vi "DUT Test.vi"(8 "error in (no error)":errorcluster, 11 "DUT cluster in":T1) -> (0 "error out":errorcluster, 3 "DUT cluster out":T1)   [LabVIEW 2018, in "Application.lvlib"]
uses:
  Application.lvlib
  DRV cluster.ctl
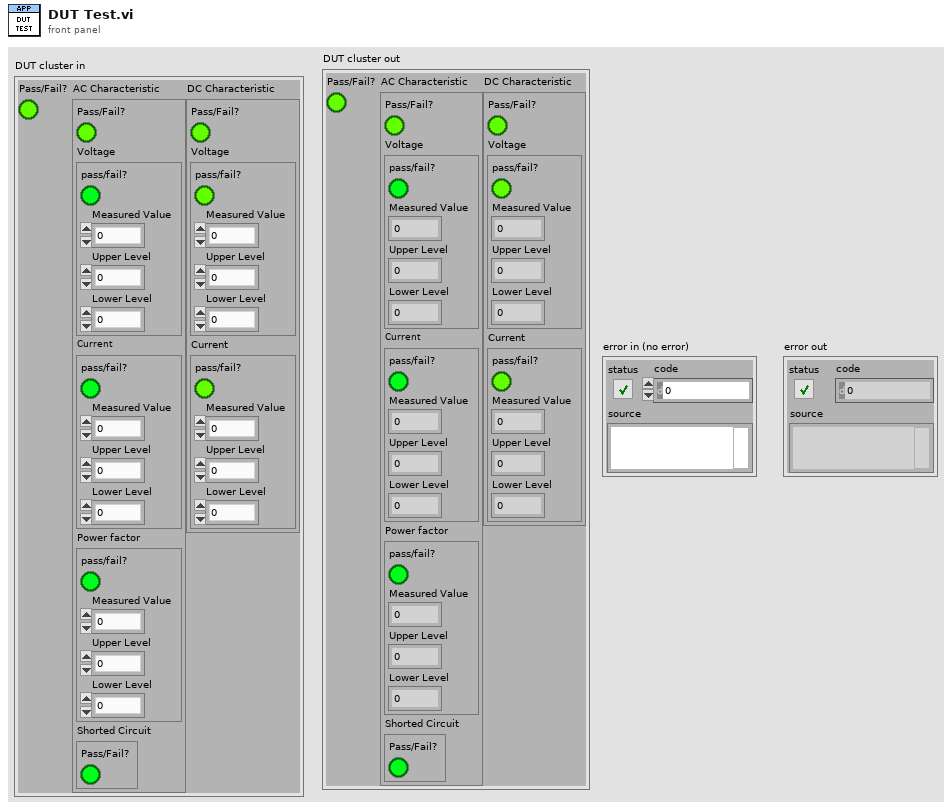
[diagram p1: front panel]
types:
  T1 = typedef "Application.lvlib/DRV cluster.ctl" = cluster{"Pass/Fail?":bool, "AC Characteristic":cluster{"Pass/Fail?":bool, "Voltage":cluster{"pass/fail?":bool, "Measured Value":dbl, "Upper Level":dbl, "Lower Level":dbl}, "Current":cluster{"pass/fail?":bool, "Measured Value":dbl, "Upper Level":dbl, "Lower Level":dbl}, "Power factor":cluster{"pass/fail?":bool, "Measured Value":dbl, "Upper Level":dbl, "Lower Level":dbl}, "Shorted Circuit":cluster{"Pass/Fail?":bool}}, "DC Characteristic":cluster{"Pass/Fail?":bool, "Voltage":cluster{"pass/fail?":bool, "Measured Value":dbl, "Upper Level":dbl, "Lower Level":dbl}, "Current":cluster{"pass/fail?":bool, "Measured Value":dbl, "Upper Level":dbl, "Lower Level":dbl}}}
  T2 = cluster{"Pass/Fail?":bool, "Voltage":cluster{"pass/fail?":bool, "Measured Value":dbl, "Upper Level":dbl, "Lower Level":dbl}, "Current":cluster{"pass/fail?":bool, "Measured Value":dbl, "Upper Level":dbl, "Lower Level":dbl}}
  T3 = cluster{"Pass/Fail?":bool, "Voltage":cluster{"pass/fail?":bool, "Measured Value":dbl, "Upper Level":dbl, "Lower Level":dbl}, "Current":cluster{"pass/fail?":bool, "Measured Value":dbl, "Upper Level":dbl, "Lower Level":dbl}, "Power factor":cluster{"pass/fail?":bool, "Measured Value":dbl, "Upper Level":dbl, "Lower Level":dbl}, "Shorted Circuit":cluster{"Pass/Fail?":bool}}
  T4 = cluster{"pass/fail?":bool, "Measured Value":dbl, "Upper Level":dbl, "Lower Level":dbl}
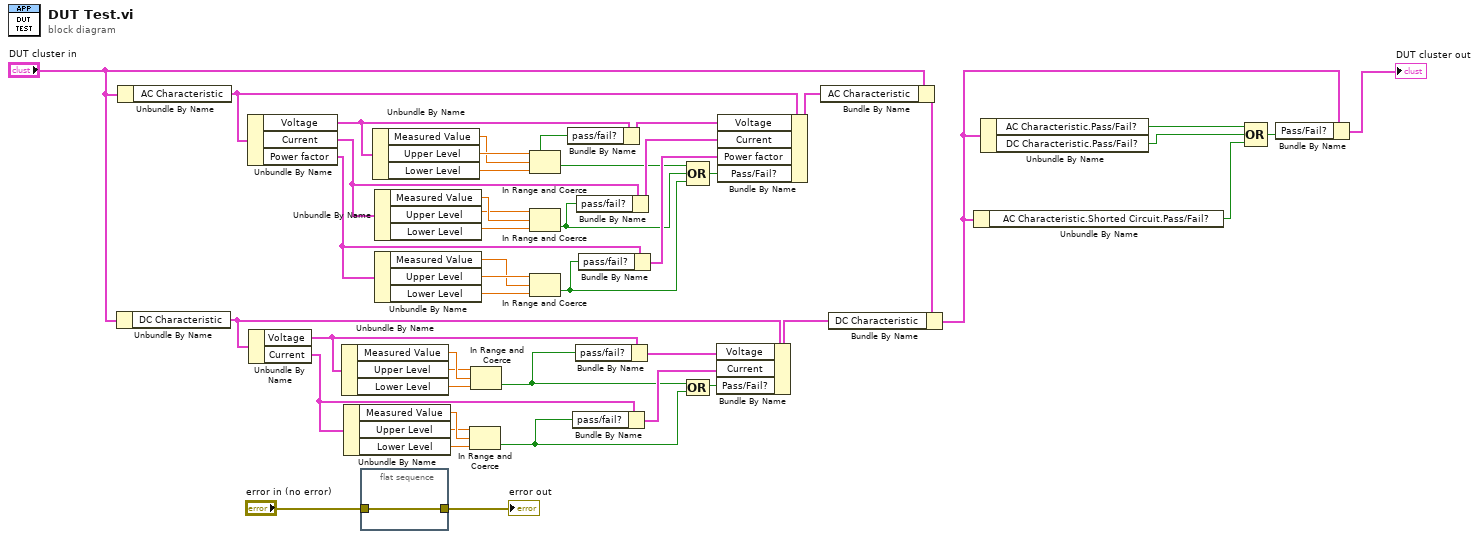
[diagram p0: block diagram]
diagram:
  n1 = Unbundle By Name("DUT cluster in") -> ("DC Characteristic"=w21:T2)
  n2 = Unbundle By Name("DUT cluster in") -> ("AC Characteristic"=w34:T3)
  n3 = Unbundle By Name(w34) -> ("Voltage"=w43:T4, "Current"=w39:T4, "Power factor"=w35:T4)
  n4 = Unbundle By Name(w21) -> ("Voltage"=w29:T4, "Current"=w22:T4)
  n5 = Unbundle By Name(w29) -> ("Measured Value"=w28:dbl, "Upper Level"=w27:dbl, "Lower Level"=w26:dbl)
  n6 = Unbundle By Name(w22) -> ("Measured Value"=w25:dbl, "Upper Level"=w24:dbl, "Lower Level"=w23:dbl)
  n7 = flat-sequence {
    tunnel: [w47] -> w5
    tunnel: "error in (no error)" -> [w47]
    frame #0 {
    }
  }
  n8 = Unbundle By Name(w43) -> ("Measured Value"=w44:dbl, "Upper Level"=w46:dbl, "Lower Level"=w45:dbl)
  n9 = Unbundle By Name(w39) -> ("Measured Value"=w42:dbl, "Upper Level"=w41:dbl, "Lower Level"=w40:dbl)
  n10 = Unbundle By Name(w35) -> ("Measured Value"=w36:dbl, "Upper Level"=w38:dbl, "Lower Level"=w37:dbl)
  n11 = In Range and Coerce(upper limit=w24, x=w25, lower limit=w23) -> (In Range?=w1:bool)  [unwired: 1 out]
  n12 = In Range and Coerce(upper limit=w27, x=w28, lower limit=w26) -> (In Range?=w6:bool)  [unwired: 1 out]
  n13 = In Range and Coerce(upper limit=w46, x=w44, lower limit=w45) -> (In Range?=w9:bool)  [unwired: 1 out]
  n14 = In Range and Coerce(upper limit=w41, x=w42, lower limit=w40) -> (In Range?=w8:bool)  [unwired: 1 out]
  n15 = In Range and Coerce(upper limit=w38, x=w36, lower limit=w37) -> (In Range?=w7:bool)  [unwired: 1 out]
  n16 = Bundle By Name(cluster=w43, "pass/fail?"=w9) -> (w10:T4)
  n17 = Bundle By Name(cluster=w22, "pass/fail?"=w1) -> (w13:T4)
  n18 = Bundle By Name(cluster=w29, "pass/fail?"=w6) -> (w14:T4)
  n19 = Bundle By Name(cluster=w39, "pass/fail?"=w8) -> (w33:T4)
  n20 = Bundle By Name(cluster=w35, "pass/fail?"=w7) -> (w32:T4)
  n21 = Compound Arithmetic op=OR(w9, w8, w7) -> (w31:bool)
  n22 = Compound Arithmetic op=OR(w6, w1) -> (w12:bool)
  n23 = Bundle By Name(cluster=w21, "Voltage"=w14, "Current"=w13, "Pass/Fail?"=w12) -> (w19:T2)
  n24 = Bundle By Name(cluster=w34, "Voltage"=w10, "Current"=w33, "Power factor"=w32, "Pass/Fail?"=w31) -> (w30:T3)
  n25 = Bundle By Name(cluster="DUT cluster in", "AC Characteristic"=w30) -> (w18:T1)
  n26 = Bundle By Name(cluster=w18, "DC Characteristic"=w19) -> (w3:T1)
  n27 = Unbundle By Name(w3) -> ("AC Characteristic.Shorted Circuit.Pass/Fail?"=w2:bool)
  n28 = Unbundle By Name(w3) -> ("AC Characteristic.Pass/Fail?"=w17:bool, "DC Characteristic.Pass/Fail?"=w16:bool)
  n29 = Compound Arithmetic op=OR(w17, w16, w2) -> (w15:bool)
  n30 = Bundle By Name(cluster=w3, "Pass/Fail?"=w15) -> (→"DUT cluster out":T1)
  "error out" <- w5
